vi "Find Oneof Field Getter.vi"(8 "error in (no error)":errorcluster, 9 "getter vi name":string, 10 "oneof container name":string, 11 "library in":refnum<vi>) -> (0 "error out":errorcluster, 1 "found?":bool, 2 "getter vi":refnum<vi>, 3 "library out":refnum<vi>)   [LabVIEW 2019, in "gRPC Template Creation Utility.lvlib"]
uses:
  gRPC Template Creation Utility.lvlib
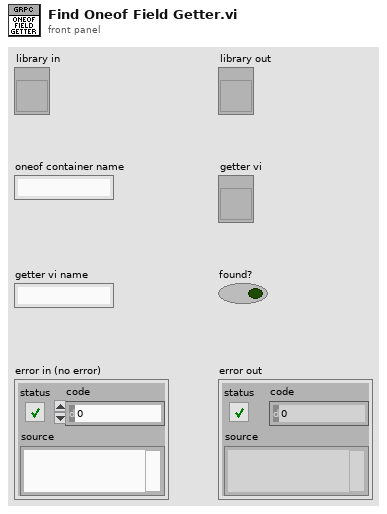
[diagram p1: front panel]
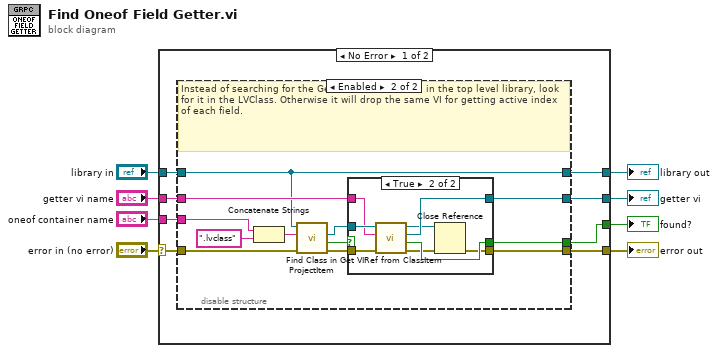
[diagram p0: block diagram]
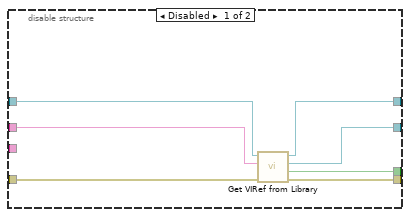
[diagram p2: hidden frame]
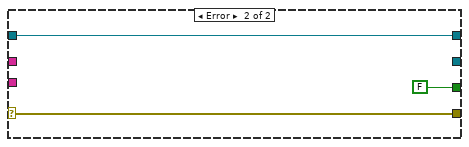
[diagram p4: hidden frame]
diagram:
  n1 = case shown="No Error" "error in (no error)" {
    selector: "error in (no error)" -> [w9 w47]
    tunnel: [w16 w45] -> w8
    tunnel: "oneof container name" -> [w15 _]
    tunnel: "library in" -> [w14 w45]
    tunnel: [w13 w47] -> w5
    tunnel: "getter vi name" -> [w12 _]
    tunnel: [w11 FALSE ("Found ?")] -> w3
    tunnel: [w10 _] -> w2
    frame No Error {
      n2 = disable-structure shown="Enabled" {
        disable-tunnel: [w23 w28] -> w10
        disable-tunnel: [w22 w27] -> w11
        disable-tunnel: w12 -> [w21 w30]
        disable-tunnel: [w20 w24] -> w16
        disable-tunnel: [w19 w26] -> w13
        disable-tunnel: w14 -> [w18 w24]
        disable-tunnel: w9 -> [w17 w25]
        disable-tunnel: w15 -> [_ w35]
        frame Disabled {
          n3 = call "Get VIRef from Library.vi"("error in (no error)"=w17, "item name"=w21, "library in"=w18) -> ("error out"=w19:errorcluster, "found"=w22:bool, "vi"=w23:refnum<vi>, "library out"=w20:refnum<vi>)  [unwired: 5 in]
        }
        frame Enabled {
          # "Instead of searching for the GetActiveFieldIndex.vi in the top level library, look for it in the LVClass. Otherwise it will drop the same VI for getting active index of each field."
          n4 = Concatenate Strings(w35, ".lvclass" ("string")) -> (w33:string)
          n5 = call "Find Class in ProjectItem.vi"("error in (no error)"=w25, "Class Name"=w33, "ProjectItem in"=w24) -> ("error out"=w29:errorcluster, "Found?"=w32:bool, "LVClass out"=w31:refnum<vi>)  [unwired: 5 in, 1 out]
          n6 = case shown="True" w32 {
            tunnel: w31 -> [_ w44]
            tunnel: w30 -> [_ w43]
            tunnel: w29 -> [w36 w42]
            tunnel: [_ w41] -> w28
            tunnel: [_ w40] -> w27
            tunnel: [w36 w37] -> w26
            frame False {
            }
            frame True {
              n7 = call "Get VIRef from ClassItem.vi"("error in (no error)"=w42, "item name"=w43, "class in"=w44) -> ("error out"=w39:errorcluster, "found"=w40:bool, "vi"=w41:refnum<vi>, "class out"=w38:refnum<vi>)  [unwired: 5 in]
              n8 = Close Reference(reference=w38, error in (no error)=w39) -> (error out=w37:errorcluster)
            }
          }
        }
      }
    }
    frame Error {
    }
  }
  "library out" <- w8
  "error out" <- w5
  "found?" <- w3
  "getter vi" <- w2
